vi "PH_Powermeter_BaseClass.PC Set Range.vi"(0 "VI in":refnum<vi>, 2 "Wanted Range":u32=1, 5 "error in (no error)":errorcluster) -> (14 "VI out":refnum<vi>, 19 "error out":errorcluster)   [LabVIEW 2014, in "PH_Powermeter_BaseClass.lvlib"]
doc: "If the incoming value is not zero and deiffers from stored value, the scaling factor is set to own attributtes. Aferwards, the energy is recalculated and set as well to own attributes as to GUI and DIM service."
uses:
  PH_Powermeter_BaseClass.lvlib
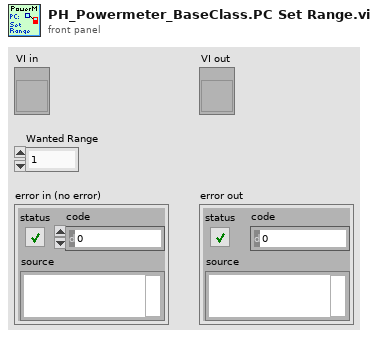
[diagram p1: front panel]
types:
  T1 = typedef "PH_Powermeter_BaseClass.lvlib/PH_Powermeter_BaseClass.i attribute.ctl" = cluster{"GUI References":T2, "Connection":T3, "Head Attributes":T5, "VISA resource":refnum<visa-resource-name>, "Energy":T6, "Service ID Energy":i32, "Wanted Settings":T7, "Current Settings":T7}
  T2 = typedef "PH_Powermeter_BaseClass.lvlib/PH_Powermeter_BaseClass.GUI Refs.ctl" = cluster{"Head Attributes":refnum<vi>, "Energy":refnum<vi>, "Connection":refnum<vi>, "VISA Resource":refnum<vi>, "Energy evolution":refnum<vi>, "Scaling Factor":refnum<vi>, "Range":refnum<vi>, "Wavelength":refnum<vi>, "Trigger Level":refnum<vi>, "Wanted Settings":refnum<vi>, "Current Settings":refnum<vi>}
  T3 = typedef "PH_Powermeter_BaseClass.lvlib/PH_Powermeter_BaseClass.Connection.ctl" = cluster{"failed checks":i8, "Timeout":bool, "Data read":string, "Failure":bool, "Error":bool, "State":T4}
  T4 = typedef "PH_Powermeter_BaseClass.lvlib/PH_Powermeter_BaseClass.State.ctl" = enum32{"off", "operating", "opened", "checked", "connected", "Sets to change", "running"}
  T5 = typedef "PH_Powermeter_BaseClass.lvlib/PH_Powermeter_BaseClass.Head Attributes.ctl" = cluster{"Instrument Type":string, "Head Version":string, "Head Name":string, "Serial Number":string, "Firmware":string, "Sensor Type":string, "MinimumRange":u32, "Maximum Range":u32, "Min Wavelength":i32, "Max Wavelength":i32}
  T6 = typedef "PH_Powermeter_BaseClass.lvlib/PH_Powermeter_BaseClass.Energy.ctl" = cluster{"current Value":dbl, "unscaled":dbl, "Scaling Factor":dbl}
  T7 = typedef "PH_Powermeter_BaseClass.lvlib/PH_gentec_BaseClass.Head Settings.ctl" = cluster{"Trigger Level":dbl, "Wavelength":u32, "Range":u32}
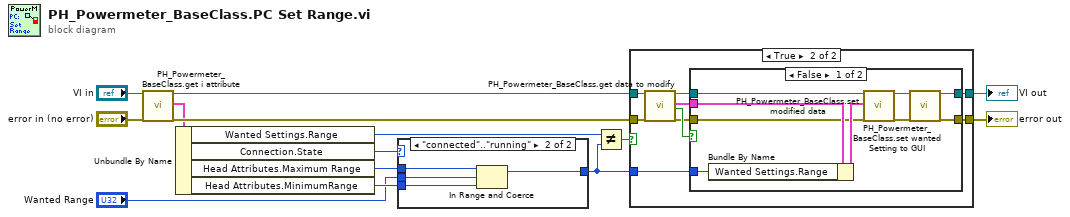
[diagram p0: block diagram]
diagram:
  n1 = call "PH_Powermeter_BaseClass.get i attribute.vi"("i ref in"="VI in", "error in (no error)"="error in (no error)") -> ("i ref out"=w9:refnum<vi>, "i attribute"=w8:T1, "error out"=w10:errorcluster)  [unwired: 15 in]
  n2 = Unbundle By Name(w8) -> ("Wanted Settings.Range"=w7:u32, "Connection.State"=w1:T4, "Head Attributes.Maximum Range"=w5:u32, "Head Attributes.MinimumRange"=w4:u32)
  n3 = case shown="\"connected\"..\"running\"" w1 {
    tunnel: w5 -> [_ w19]
    tunnel: w4 -> [_ w18]
    tunnel: "Wanted Range" -> [w15 w17]
    tunnel: [w15 w16] -> w2
    frame "off", Default {
    }
    frame "connected".."running" {
      n4 = In Range and Coerce(upper limit=w19, x=w17, lower limit=w18) -> (coerced(x)=w16:u32)  [unwired: 1 out]
    }
  }
  n5 = Not Equal?(x=w7, y=w2) -> (x != y?=w6:bool)
  n6 = case shown="True" w6 {
    tunnel: [w20 w28] -> w14
    tunnel: [w21 w26] -> w12
    tunnel: w10 -> [w20 w24]
    tunnel: w9 -> [w21 w23]
    tunnel: w2 -> [_ w22]
    frame False {
    }
    frame True {
      n7 = call "PH_Powermeter_BaseClass.get data to modify.vi"("i ref in"=w23, "error in (no error)"=w24) -> ("i ref out"=w25:refnum<vi>, "i attribute"=w30:T1, "timed out"=w29:bool, "error out"=w27:errorcluster)  [unwired: 14 in]
      n8 = case shown="False" w29 {
        tunnel: w25 -> [w39 w41]
        tunnel: [w31 w41] -> w26
        tunnel: w27 -> [w35 w40]
        tunnel: [w33 w40] -> w28
        tunnel: w30 -> [w37 _]
        tunnel: w22 -> [w36 _]
        frame False {
          n9 = Bundle By Name(cluster=w37, "Wanted Settings.Range"=w36) -> (w38:T1)
          n10 = call "PH_Powermeter_BaseClass.set modified data.vi"("i ref in"=w39, "i attribute"=w38, "error in (no error)"=w35) -> ("i ref out"=w32:refnum<vi>, "error out"=w34:errorcluster)  [unwired: 15 in]
          n11 = call "PH_Powermeter_BaseClass.set wanted Setting to GUI.vi"("VI in"=w32, "error in (no error)"=w34) -> ("VI out"=w31:refnum<vi>, "error out"=w33:errorcluster)  [unwired: 16 in]
        }
        frame True {
        }
      }
    }
  }
  "error out" <- w14
  "VI out" <- w12
